vi "myRIO_BRig_RT_dataLC_Wrong_Probability_l1.vi"() -> (2 "output_Wrong_Probability_l1":i32)   [LabVIEW 2014]
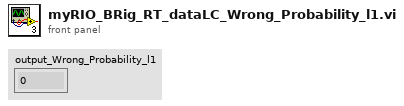
[diagram p1: front panel]
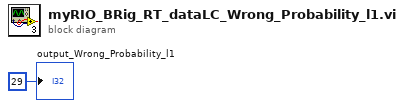
[diagram p0: block diagram]
diagram:
  "output_Wrong_Probability_l1" <- 29 ("output_iBlock")
